vi "CNR_ConvertImageTo1DArray.vi"(8 "error in (no error)":errorcluster, 11 "Refnum in":T1) -> (0 "error out":errorcluster, 3 "Array":dbl[](array[numeric]))   [LabVIEW 2023]
uses:
  <vilib>/vision/Image Controls.llb/IMAQ Image.ctl
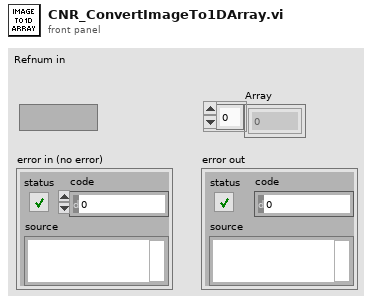
[diagram p1: front panel]
types:
  T1 = typedef "IMAQ Image.ctl" = refnum<image>
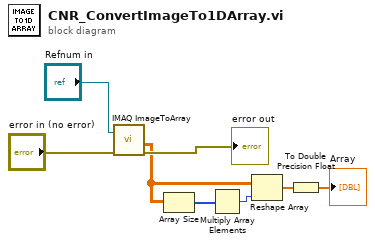
[diagram p0: block diagram]
diagram:
  n1 = call "IMAQ ImageToArray"("error in (no error)"="error in (no error)", "Image"="Refnum in") -> ("Image Pixels (Float)"=w1:sgl[][], "error out"=→"error out":errorcluster)  [unwired: 2 in, 3 out]
  n2 = Array Size(array=w1) -> (size(s)=w5:i32[])
  n3 = Multiply Array Elements(1:w5) -> (0:w3:i32)
  n4 = Reshape Array(w1, w3) -> (w2:sgl[])
  n5 = To Double Precision Float(number=w2) -> (double precision float=→"Array":dbl[])
